vi "Interpret Joysticks.vi"(10 "Joystick Controls":T13) -> (0 "Vanna Teleop Command":T7, 1 "Intake Teleop Command":T4, 2 "Climb Teleop Command":T9, 3 "Drive Teleop command":T11, 4 "Index Teleop Command":dbl, 5 "Shoot Teleop Command":T1)   [LabVIEW 2019]
uses:
  Joystick Controls.ctl
  Drive/Drive Command Typedef.ctl
  Drive/Drive Mode Typedef.ctl
  Climb/Climb Command Type Def.ctl
  Climb/Climb Mode Type Def.ctl
  Vanna/Vanna Command Type Def.ctl
  Vanna/Vanna Mode Type Def.ctl
  Intake/Intake Command Type Def.ctl
  Intake/Intake Mode Type Def.ctl
  <vilib>/Rock Robotics/WPI/Solenoid/WPI_SolenoidValue.ctl
  Shoot/Shooter Command Type Def.ctl
  Shoot/Shooter Mode Type Def.ctl
  Shoot/Shooter Preset speeds Type Def.ctl
panel:
  # "NOT COMPLETE YET, BUT INTENDED CONTROLS: \n\nDRIVER JOYSTICK\nTwo Joysticks for driving (Left Y is throttle, Right X is turn)\nTriggers for intaking. Pressing all the way forces a retract/extend. Keeping them less than 75% leaves the pheumatic state alone. May make speed on/off, not continuous\nLeft bumper: turbo drive\nRight Bumper: auto-align\n\nOPERATOR JOYSTICK\nDPAD: UP/Down = climber up/down\nDPAD Sideways = Skywalker manual\nLeft Bumper = Skywalker auto (gyroscope)\nY Button: Auto range shooter\nA, B, X buttons: preset speeds shooter\nRight joystick X: Vanna Manual. must have deadband.\nLeft Joystick Y: UP = Rotation control; DOWN = position control\nVanna pops up whenever its not disabled\nRight Trigger: Fire Ball (Run indexer)\nLeft Trigger: Change shooter angle"
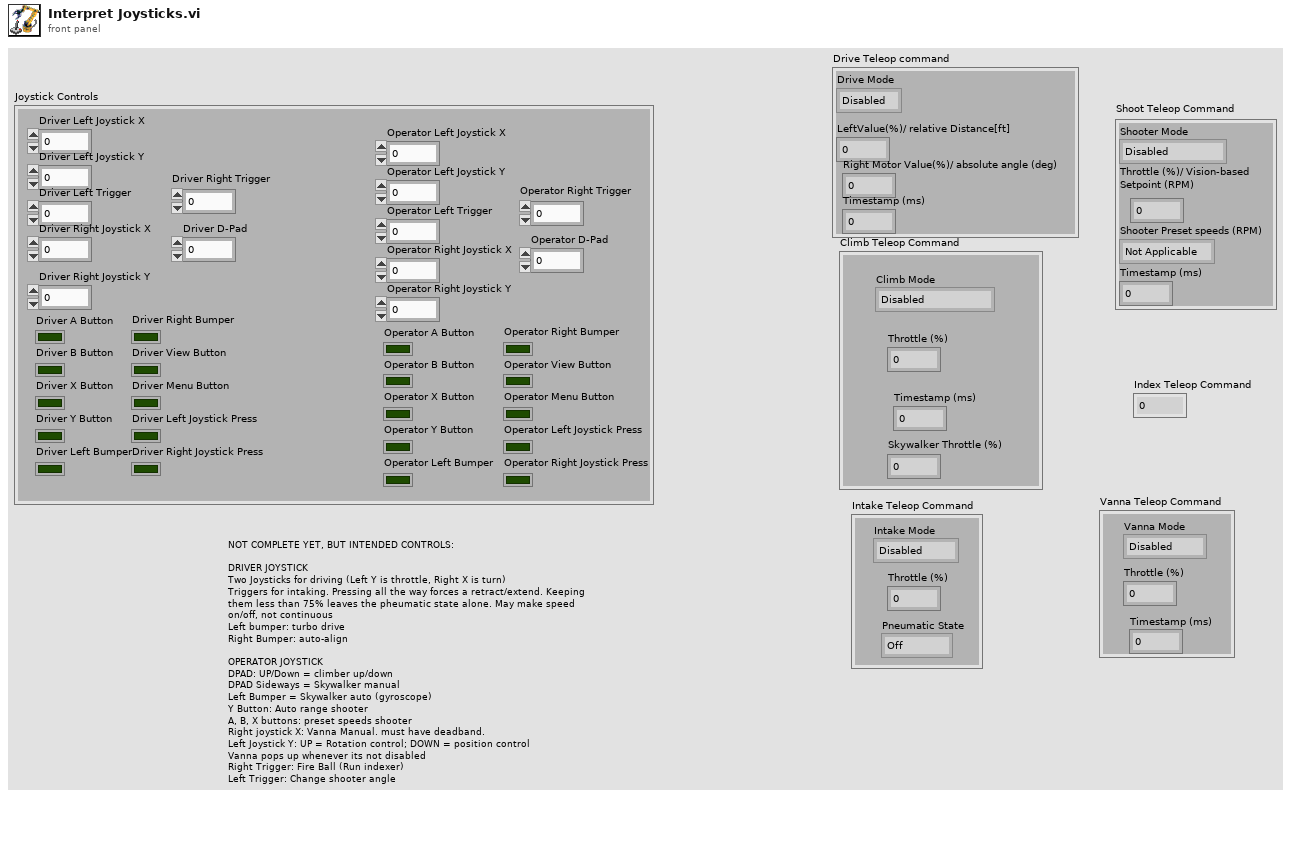
[diagram p1: front panel]
types:
  T1 = typedef "Shooter Command Type Def.ctl" = cluster{"Shooter Mode":T2, "Throttle (%)/ Vision-based\nSetpoint (RPM)":dbl, "Shooter Preset speeds (RPM)":T3, "Timestamp (ms)":dbl}
  T2 = typedef "Shooter Mode Type Def.ctl" = enum16{"Disabled", "Raw Throttle", "Preset Velocity Control", "Vision-based Velocity Control"}
  T3 = typedef "Shooter Preset speeds Type Def.ctl" = enum16{"Not Applicable", "Target Zone", "Initiation Line", "Close end of Trench Run", "Control Panel"}
  T4 = typedef "Intake Command Type Def.ctl" = cluster{"Intake Mode":T5, "Throttle (%)":dbl, "Pneumatic State":T6}
  T5 = typedef "Intake Mode Type Def.ctl" = enum16{"Disabled", "Enabled"}
  T6 = typedef "WPI_SolenoidValue.ctl" = enum16{"Off", "On", "Forward", "Reverse"}
  T7 = typedef "Vanna Command Type Def.ctl" = cluster{"Vanna Mode":T8, "Throttle (%)":dbl, "Timestamp (ms)":dbl}
  T8 = typedef "Vanna Mode Type Def.ctl" = enum16{"Disabled", "Raw Throttle", "Rotation Control", "Position Control"}
  T9 = typedef "Climb Command Type Def.ctl" = cluster{"Climb Mode":T10, "Throttle (%)":dbl, "Timestamp (ms)":dbl, "Skywalker Throttle (%)":dbl}
  T10 = typedef "Climb Mode Type Def.ctl" = enum16{"Disabled", "Raw Throttle"}
  T11 = typedef "Drive Command Typedef.ctl" = cluster{"Drive Mode":T12, "LeftValue(%)/ relative Distance[ft]":dbl, "Right Motor Value(%)/ absolute angle (deg)":dbl, "Timestamp (ms)":dbl}
  T12 = typedef "Drive Mode Typedef.ctl" = enum16{"Disabled", "Auto-align", "Drive Distance", "Turn to angle", "Driver", "Driver Velocity Control"}
  T13 = typedef "Joystick Controls.ctl" = cluster{"Driver Left Joystick X":dbl, "Driver Left Joystick Y":dbl, "Driver A Button":bool, "Driver B Button":bool, "Driver X Button":bool, "Driver Y Button":bool, "Driver Left Bumper":bool, "Driver Right Bumper":bool, "Driver View Button":bool, "Driver Menu Button":bool, "Driver Left Joystick Press":bool, "Driver Right Joystick Press":bool, "Driver Left Trigger":dbl, "Driver Right Joystick X":dbl, "Driver Right Joystick Y":dbl, "Driver Right Trigger":dbl, "Operator Left Joystick X":dbl, "Operator Left Joystick Y":dbl, "Operator A Button":bool, "Operator B Button":bool, "Operator X Button":bool, "Operator Y Button":bool, "Operator Left Bumper":bool, "Operator Right Bumper":bool, "Operator View Button":bool, "Operator Menu Button":bool, "Operator Left Joystick Press":bool, "Operator Right Joystick Press":bool, "Operator Left Trigger":dbl, "Operator Right Joystick X":dbl, "Operator Right Joystick Y":dbl, "Operator Right Trigger":dbl, "Driver D-Pad":i16, "Operator D-Pad":i16}
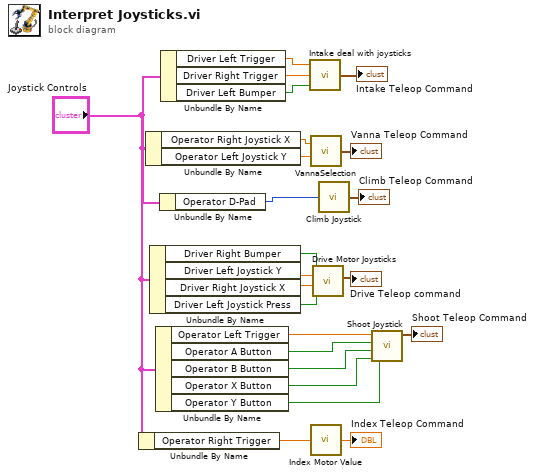
[diagram p0: block diagram]
diagram:
  n1 = Unbundle By Name("Joystick Controls") -> ("Operator Right Trigger"=w7:dbl)
  n2 = Unbundle By Name("Joystick Controls") -> ("Operator Right Joystick X"=w10:dbl, "Operator Left Joystick Y"=w9:dbl)
  n3 = Unbundle By Name("Joystick Controls") -> ("Driver Right Bumper"=w8:bool, "Driver Left Joystick Y"=w22:dbl, "Driver Right Joystick X"=w23:dbl, "Driver Left Joystick Press"=w21:bool)
  n4 = Unbundle By Name("Joystick Controls") -> ("Operator Left Trigger"=w15:dbl, "Operator A Button"=w13:bool, "Operator B Button"=w12:bool, "Operator X Button"=w11:bool, "Operator Y Button"=w6:bool)
  n5 = Unbundle By Name("Joystick Controls") -> ("Operator D-Pad"=w5:i16)
  n6 = Unbundle By Name("Joystick Controls") -> ("Driver Left Trigger"=w3:dbl, "Driver Right Trigger"=w2:dbl, "Driver Left Bumper"=w1:bool)
  n7 = call "Intake deal with joysticks.vi"("Extend?"=w1, "Negative Throttle (%)"=w2, "Positive Throttle (%)"=w3) -> ("Intake Teleop Command"=→"Intake Teleop Command":T4)
  n8 = call "VannaSelection.vi"("Rotation/position selector: Rot is neg, Pos is positive"=w9, "Vanna Raw throttle (%)"=w10) -> ("Vanna Teleop Command"=→"Vanna Teleop Command":T7)
  n9 = call "Index Motor Value.vi"("Feed Into Shooter?"=w7) -> ("Index Teleop Command"=→"Index Teleop Command":dbl)
  n10 = call "Drive Motor Joysticks.vi"("Boost?"=w21, "Turn"=w23, "Throttle"=w22, "Auto-Align?"=w8) -> ("Teleop Drive command"=→"Drive Teleop command":T11)  [unwired: 7 in]
  n11 = call "Climb Joystick.vi"("Operator D-Pad"=w5) -> ("Climb Teleop Command"=→"Climb Teleop Command":T9)  [unwired: 2 in]
  n12 = call "Shoot Joystick.vi"("Auto Calculate Speed"=w6, "Trench Speed"=w11, "Init LIne Speed"=w12, "Target Zone Speed"=w13, "Raw Throttle"=w15) -> ("Shoot Teleop Command"=→"Shoot Teleop Command":T1)  [unwired: 6 in]
